vi "Set_Parameter_Instrument (Json).vi"(8 "error in (no error)":errorcluster caption="entrée d'erreur (pas d'erreur)", 10 "Parameter (Json)":string, 11 "Wait_Frame_ERP1 en entrée":refnum<class "Wait_Frame_ERP1.lvclass">) -> (0 "error out":errorcluster caption="sortie d'erreur", 3 "Wait_Frame_ERP1 en sortie":refnum<class "Wait_Frame_ERP1.lvclass">)   [LabVIEW 2020, in "Library Test.lvlib" / "Wait_Frame_ERP1.lvclass"]
uses:
  Wait_Frame_ERP1.lvclass
  C:/Users/ngarcin/OneDrive - Altyor/Standard TB/Class/Test/Test (Default)/Test (Default).lvclass
  Wait_Frame_ERP1.lvclass/Wait_Frame_ERP1.ctl
  JSON API/JSON Value/Set from JSON string.vi
  Test_Wtih_Instr/Test_With_Inst.lvclass
  JSON API/JSON Value/JSON Value.lvclass
  JSON API/Variant JSON/Variant JSON.lvlib
  JSON API/Get Polymorphic/JSON GetSet.lvlib
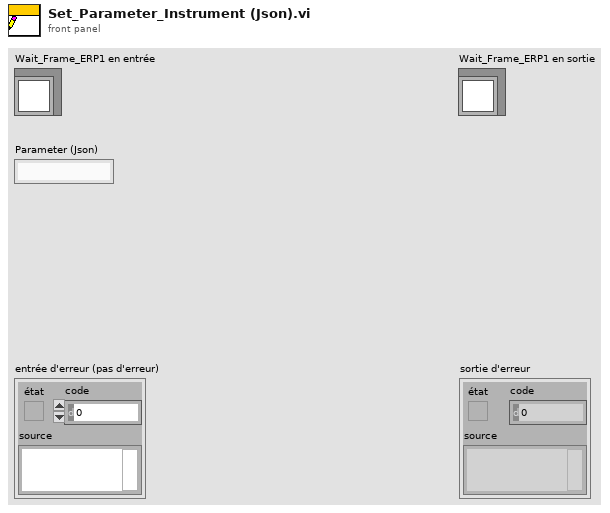
[diagram p1: front panel]
types:
  T1 = cluster{"TimeOut":u16, "R-org":string, "Frame Type":enum16{"Teach IN", "Normal Mode"}}
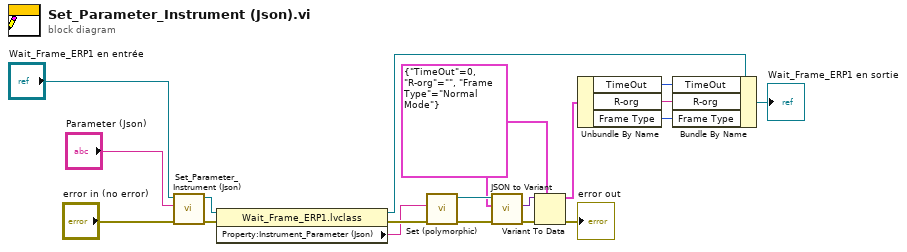
[diagram p0: block diagram]
diagram:
  w3 = T1 {"TimeOut"=0, "R-org"="", "Frame Type"=enum."Normal Mode"}
  n1 = call-parent "Set_Parameter_Instrument (Json).vi"("error in (no error)"="error in (no error)", "Parameter (Json)"="Parameter (Json)", "Test (Default) en entrée"="Wait_Frame_ERP1 en entrée") -> ("error out"=w15:errorcluster, "Test (Default) en sortie"=w16:refnum<class "Wait_Frame_ERP1.lvclass">)  [unwired: 7 in]
  n2 = property class="Wait_Frame_ERP1.lvclass"(reference=w16, error in=w15) -> (reference out=w8:refnum<class "Wait_Frame_ERP1.lvclass">, error out=w10:errorcluster, "Property:Instrument_Parameter (Json)"=w9:string)
  n3 = call-poly "Set (polymorphic).vi"("error in (no error)"=w10, "JSON stream"=w9) -> ("error out"=w12:errorcluster, "JSON Value out"=w14:refnum<class "JSON Value.lvclass">)  [unwired: 7 in, 1 out]
  n4 = call "JSON to Variant.vi"("error in (no error)"=w12, "Variant (Data Type)"=w3, "JSON Value"=w14) -> ("error out"=w13:errorcluster, "Variant out"=w11:variant)  [unwired: 7 in]
  n5 = Variant To Data(error in=w13, type=w3, Variant=w11) -> (data=w7:T1, error out=→"error out":errorcluster)
  n6 = Unbundle By Name(w7) -> ("TimeOut"=w6:u16, "R-org"=w5:string, "Frame Type"=w1:enum16{"Teach IN", "Normal Mode"})
  n7 = Bundle By Name(cluster=w8, "TimeOut"=w6, "R-org"=w5, "Frame Type"=w1) -> (→"Wait_Frame_ERP1 en sortie":refnum<class "Wait_Frame_ERP1.lvclass">)
